vi "Smith Multi Plot with Styles.vi"() -> ()   [LabVIEW 2023]
doc: "Uses the Smith Multi Plot VI and the Normalize Smith Plot VI to draw multiple smith plots in a picture indicator. This example demonstrates the line styles available, as well as how to normalize data for display."
panel:
  in  "Style 2":u16(ring)=1 items=["Points", "Lines", "Points & Lines"]
  in  "Color 2":u32(colorbox)=16777113
  in  "Style 1":u16(ring)=2 items=["Points", "Lines", "Points & Lines"]
  in  "Color 1":u32(colorbox)=52479
  in  "Autoscale?":bool
  out "Smith Plot":picture
  # "Overview: Uses the Smith Plot VI to draw a smith plot in a picture indicator.\nInstructions:\n1. Run the VI.\n2. Change the color and style controls to view the different cosmetic styles.\n3. Toggle the Autoscale? control to switch between autoscaling and showing the entire plot and run the VI again."
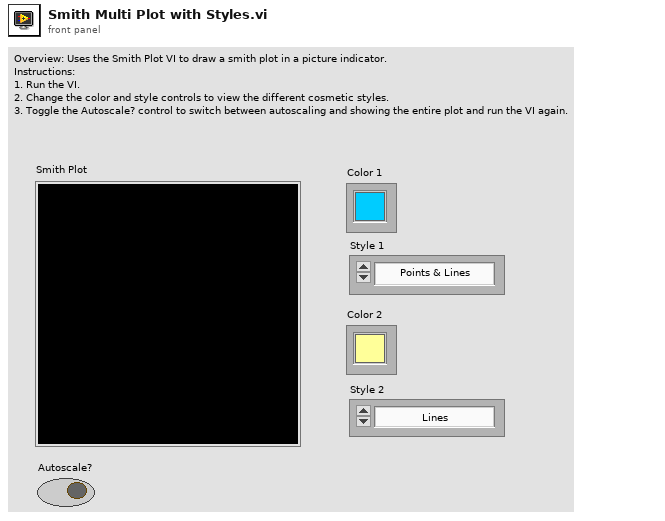
[diagram p1: front panel]
types:
  T1 = cluster{"normalized smith points {r,x}":cluster{"r":dbl, "x":dbl}[]}[]
  T2 = cluster{"Style 1":u16, "Color 1":u32, "Color 1":u32}
  T3 = cluster{"Style 2":u16, "Color 2":u32, "Color 2":u32}
  T4 = cluster{"Style 2":u16, "Color 2":u32, "Color 2":u32}[]
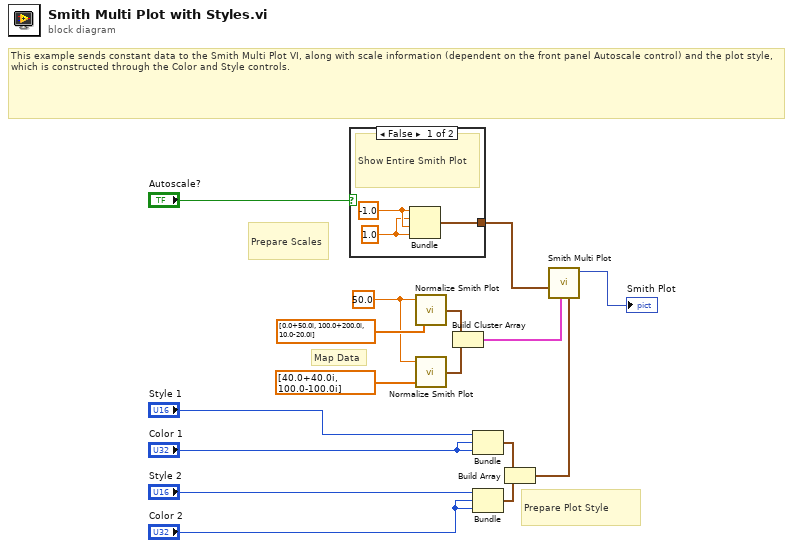
[diagram p0: block diagram]
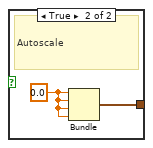
[diagram p2: hidden frame]
diagram:
  w1 = 50.0
  # "This example sends constant data to the Smith Multi Plot VI, along with scale information (dependent on the front panel Autoscale control) and the plot style, which is constructed through the Color and Style controls."
  # "Prepare Plot Style"
  # "Map Data"
  # "Prepare Scales"
  n1 = case shown="False" "Autoscale?" {
    tunnel: [w18 w21] -> w2
    frame False {
      w17 = 1.0
      w19 = -1.0
      # "Show Entire Smith Plot"
      n2 = Bundle(w19, w17, w19, w17) -> (w18:cluster{dbl, dbl, dbl, dbl})  [unwired: 1 in]
    }
    frame True {
      w20 = 0.0
      # "Autoscale"
      n3 = Bundle(w20, w20, w20, w20) -> (w21:cluster{dbl, dbl, dbl, dbl})  [unwired: 1 in]
    }
  }
  n4 = call <vilib>:"Normalize Smith Plot.vi"("points complex"=cdb[] [0.0+50.0i, 100.0+200.0i, 10.0-20.0i] ("Plot 1"), "Zo (50.0)"=w1) -> ("normalized smith points {r,x}"=w15:cluster{"r":dbl, "x":dbl}[])  [unwired: 1 in]
  n5 = call <vilib>:"Normalize Smith Plot.vi"("points complex"=cdb[] [40.0+40.0i, 100.0-100.0i] ("Plot 2"), "Zo (50.0)"=w1) -> ("normalized smith points {r,x}"=w14:cluster{"r":dbl, "x":dbl}[])  [unwired: 1 in]
  n6 = Build Cluster Array(w15, w14) -> (w13:T1)
  n7 = Bundle("Style 1"="Style 1", "Color 1"="Color 1", "Color 1"="Color 1") -> (w10:T2)  [unwired: 1 in]
  n8 = Bundle("Style 2"="Style 2", "Color 2"="Color 2", "Color 2"="Color 2") -> (w9:T3)  [unwired: 1 in]
  n9 = Build Array(w10, w9) -> (w8:T4)
  n10 = call <vilib>:"Smith Multi Plot.vi"("smith plot cosmetics"=w8, "smith multi plot"=w13, "smith plot section"=w2) -> ("new picture"=→"Smith Plot":picture)  [unwired: 8 in]
